vi "Close File.vi"(8 "error in":errorcluster, 11 "TDMS in":refnum<class "TDMS.lvclass">) -> (0 "error out":errorcluster, 3 "TDMS out":refnum<class "TDMS.lvclass">)   [LabVIEW 2020, in "Manejador archivo.lvlib" / "TDMS.lvclass"]
uses:
  TDMS.lvclass
  TDMS.lvclass/TDMS.ctl
  Read tdms file ref.vi
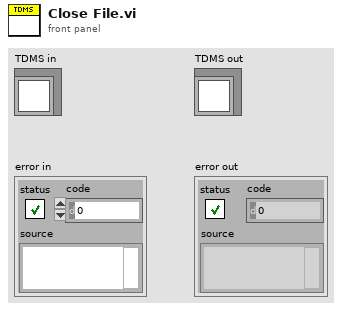
[diagram p1: front panel]
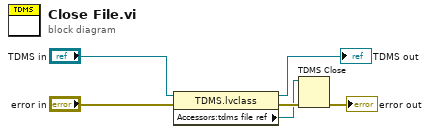
[diagram p0: block diagram]
diagram:
  n1 = property class="TDMS.lvclass"(reference="TDMS in", error in="error in") -> (reference out=→"TDMS out":refnum<class "TDMS.lvclass">, error out=w4:errorcluster, "Accessors:tdms file ref"=w2:refnum<k34>)
  n2 = TDMS Close(8:w4, 11:w2) -> (0:→"error out":errorcluster)  [unwired: 1 out]
